vi "L0_SumnAdds_File_Create.vi"(1 "input cluster":T1, 2 "Serial Number":string="testFile") -> (0 "appended path":path)   [LabVIEW 2009]
uses:
  <vilib>/Utility/NIReport.llb/NI_report.lvclass
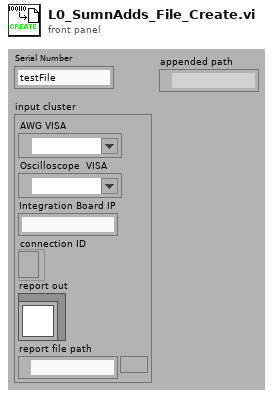
[diagram p1: front panel]
types:
  T1 = cluster{"AWG VISA":refnum<visa-resource-name>, "Oscilloscope  VISA ":refnum<visa-resource-name>, "Integration Board IP":string, "connection ID":refnum<k5>, "report out":refnum<class "NI_report.lvclass">, "report file path":path}
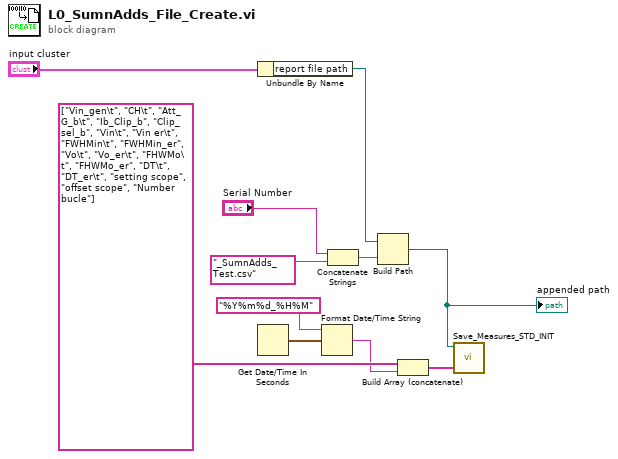
[diagram p0: block diagram]
diagram:
  n1 = Unbundle By Name("input cluster") -> ("report file path"=w4:path)
  n2 = Get Date/Time In Seconds() -> (seconds since 1Jan1904=w9:timestamp)
  n3 = Format Date/Time String(time format string (%c)="%Y%m%d_%H%M", seconds (now)=w9) -> (date/time string=w7:string)  [unwired: 1 in]
  n4 = Concatenate Strings("Serial Number", "_SumnAdds_Test.csv" ("format string")) -> (w5:string)
  n5 = Build Path(base path=w4, name or relative path=w5) -> (appended path=w2:path)
  "appended path" <- w2
  n6 = Build Array (concatenate)(string[] ["Vin_gen\t", "CH\t", "Att_G_b\t", "Ib_Clip_b", "Clip_sel_b", "Vin\t", "Vin er\t", "FWHMin\t", "FWHMin_er", "Vo\t", "Vo_er\t", "FHWMo\t", "FHWMo_er", "DT\t", "DT_er\t", "setting scope", "offset scope", "Number bucle"] ("appended array"), w7) -> (w10:string[])
  n7 = call "Save_Measures_STD_INIT.vi"("appended array"=w10, "file path (dialog if empty)"=w2) -> ()  [unwired: 10 in]
